vi "AngularDistance.vi"(2 "Goal Angle (deg) [0,360]":dbl format="%#_13g", 3 "Current Angle (deg) [-Inf,+Inf]":dbl format="%#_13g") -> (0 "Alternate Signed Angular Distance (deg) [-360,+360]":dbl format="%_4g", 1 "Signed Angular Distance (deg) [-180,+180]":dbl format="%_4g")   [LabVIEW 2020]
doc: "Calculates the shortest signed angular distance from the Current Angle to the Goal Angle. The Goal Angle must be on [0,360] while the Current angle can be on [-Inf,+Inf]. The Alternate Signed Angular Distance is the angle in the opposite direction and is on [-360,+360]."
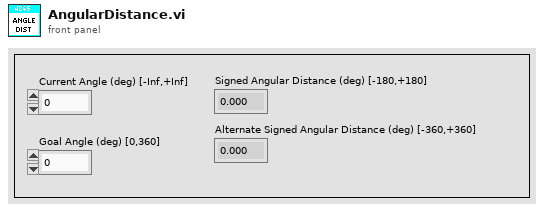
[diagram p1: front panel]
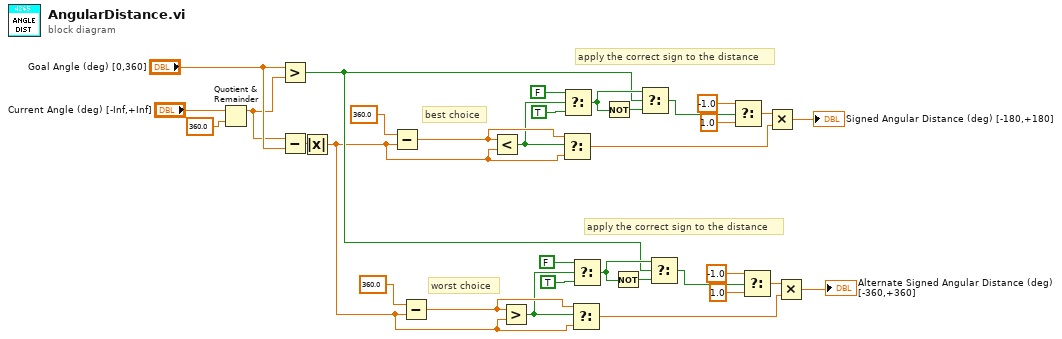
[diagram p0: block diagram]
diagram:
  # "worst choice"
  # "best choice"
  # "apply the correct sign to the distance"
  # "apply the correct sign to the distance"
  n1 = Quotient & Remainder(x="Current Angle (deg) [-Inf,+Inf]", y=360.0) -> (x-y*floor(x/y)=w28:dbl)  [unwired: 1 out]
  n2 = Greater?(x="Goal Angle (deg) [0,360]", y=w28) -> (0:w3:bool)
  n3 = Subtract(x=w28, y="Goal Angle (deg) [0,360]") -> (x-y=w31:dbl)
  n4 = Absolute Value(x=w31) -> (abs(x)=w2:dbl)
  n5 = Subtract(x=360.0, y=w2) -> (x-y=w27:dbl)
  n6 = Subtract(x=360.0, y=w2) -> (x-y=w14:dbl)
  n7 = Less?(x=w27, y=w2) -> (x < y?=w26:bool)
  n8 = Greater?(x=w14, y=w2) -> (0:w13:bool)
  n9 = Select(t=w27, s=w26, f=w2) -> (s? t:f=w17:dbl)
  n10 = Select(t=FALSE, s=w26, f=TRUE) -> (s? t:f=w23:bool)
  n11 = Select(t=w14, s=w13, f=w2) -> (s? t:f=w4:dbl)
  n12 = Select(t=FALSE, s=w13, f=TRUE) -> (s? t:f=w10:bool)
  n13 = Not(x=w23) -> (.not. x?=w22:bool)
  n14 = Not(x=w10) -> (.not. x?=w9:bool)
  n15 = Select(t=w23, s=w3, f=w22) -> (s? t:f=w21:bool)
  n16 = Select(t=w10, s=w3, f=w9) -> (s? t:f=w8:bool)
  n17 = Select(t=-1.0, s=w21, f=1.0) -> (s? t:f=w18:dbl)
  n18 = Select(t=-1.0, s=w8, f=1.0) -> (s? t:f=w5:dbl)
  n19 = Multiply(x=w18, y=w17) -> (x*y=→"Signed Angular Distance (deg) [-180,+180]":dbl)
  n20 = Multiply(x=w5, y=w4) -> (x*y=→"Alternate Signed Angular Distance (deg) [-360,+360]":dbl)
